vi "Copy Buffer to Image (ARGB).vi"(7 "Buffer Layout":T2, 8 "error in (no error)":errorcluster, 10 "ARGB Image Destination in":T1, 11 "Buffer":u8[](array[numeric])) -> (0 "error out":errorcluster, 3 "ARGB Image Destination":T1)   [LabVIEW 2020, in "image.lvlib"]
doc: "Copy the Buffer into the Image Destination.\n\nThe Destination will be resized to acommodate the Buffer's data."
uses:
  Buffer Information.ctl
  Raw Memory Information Dimension.ctl
  ARGB Image.ctl
  f11fe23a-4bac-4ce6-b593-80dfc143e0fd.vi
  <vilib>/Utility/error.llb/Error Cluster From Error Code.vi
  image.lvlib
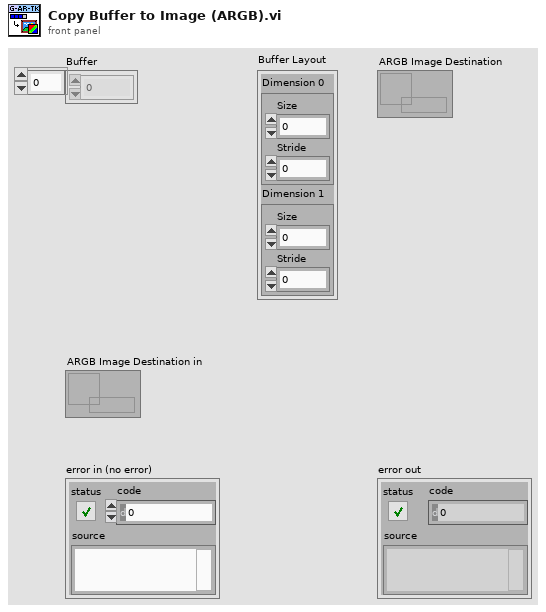
[diagram p1: front panel]
types:
  T1 = typedef "image.lvlib/ARGB Image.ctl" = refnum<data-value>
  T2 = typedef "image.lvlib/Buffer Information.ctl" = cluster{"Dimension 0":T3, "Dimension 1":T3}
  T3 = typedef "image.lvlib/Raw Memory Information Dimension.ctl" = cluster{"Size":u16, "Stride":u32}
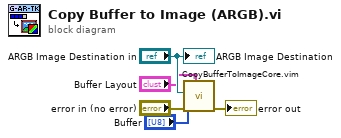
[diagram p0: block diagram]
diagram:
  n1 = call "CopyBufferToImageCore.vim"("Buffer Information"="Buffer Layout", "error in (no error)"="error in (no error)", "Dst"="ARGB Image Destination in", "Buffer"="Buffer") -> ("error out"=→"error out":errorcluster)  [unwired: 7 in]
  "ARGB Image Destination" <- "ARGB Image Destination in"
